vi "GetOrignal.vi"(3 "element":T1 {"Contours"."Type" items=["No Selection", "Point", "Line", "Rectangle", "Oval", "Polygon", "Freehand Region", "Annulus", "Unused2", "Unused3", "Broken Line", "Freehand Line", "Rotated Rectangle"]}) -> (1 "Orignal":cluster{i32, i32})   [LabVIEW 2014]
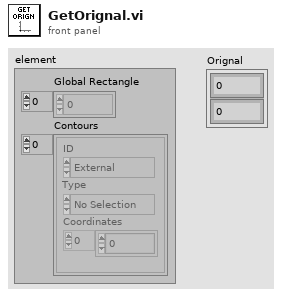
[diagram p1: front panel]
types:
  T1 = typedef "ROI Descriptor" = cluster{"Global Rectangle":i32[], "Contours":cluster{"ID":enum32{"External", "Internal"}, "Type":u32, "Coordinates":i32[]}[]}
  T2 = cluster{"ID":enum32{"External", "Internal"}, "Type":u32, "Coordinates":i32[]}[]
  T3 = cluster{"ID":enum32{"External", "Internal"}, "Type":u32, "Coordinates":i32[]}
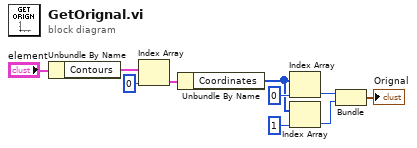
[diagram p0: block diagram]
diagram:
  n1 = Unbundle By Name("element") -> ("Contours"=w8:T2)
  n2 = Index Array(array=w8, index=0) -> (element=w7:T3)
  n3 = Unbundle By Name(w7) -> ("Coordinates"=w3:i32[])
  n4 = Index Array(array=w3, index=0) -> (element=w2:i32)
  n5 = Index Array(array=w3, index=1) -> (element=w4:i32)
  n6 = Bundle(w2, w4) -> (→"Orignal":cluster{i32, i32})  [unwired: 1 in]
